vi "clone.vi"(0 "reference":refnum<class "Graphics.lvclass">, 5 "error in (no error)":errorcluster) -> (14 "reference out":refnum<class "Graphics.lvclass">, 15 "clonedObjectRef":refnum<class "Graphics.lvclass">, 19 "error out":errorcluster)   [LabVIEW 2014, in "Graphics.lvclass"]
doc: "Clopned the object"
uses:
  <resource>/Framework/Providers/Open_GDS/UML/Graphics_class/Graphics.lvclass
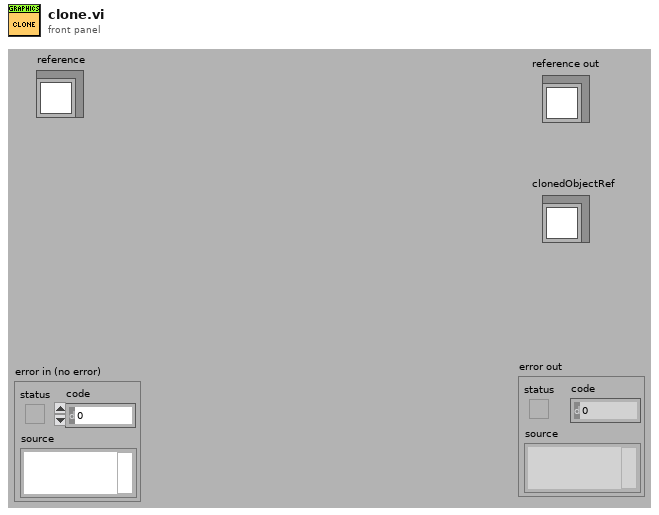
[diagram p1: front panel]
types:
  T1 = typedef "Graphics.lvclass/ObjectAttributes.ctl" = cluster{"drawColor":u32, "backgroundColor":u32, "font":T2, "fontType":T3, "picture":picture, "stroke":T4, "scaleX":dbl, "scaleY":dbl, "screenRef":refnum<vi>, "offsetX":dbl, "offsetY":dbl}
  T2 = typedef "Graphics.lvclass/FontType.ctl" = cluster{"Font Name:":string, "Size":i16, "Strikeout?":bool, "Italic?":bool, "Underline?":bool, "Outline?":bool, "Shadow?":bool, "Bold?":bool}
  T3 = typedef "Graphics.lvclass/LvFontType.ctl" = enum16{"User-specified Font", "Application Font", "System Font", "Dialog Font"}
  T4 = typedef "Graphics.lvclass/StrokeType.ctl" = enum16{"USE_DEFAULT", "SOLID", "DOTTED"}
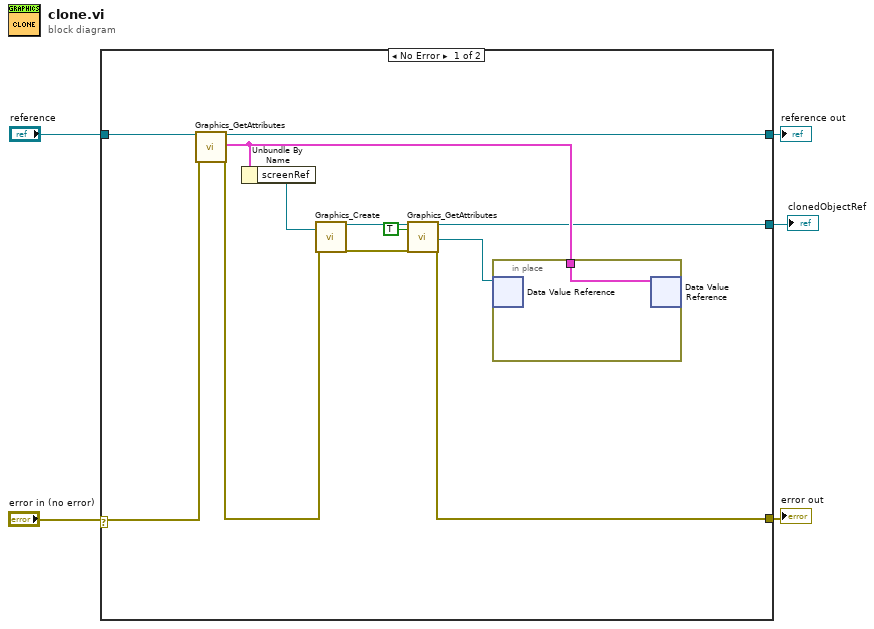
[diagram p0: block diagram]
diagram:
  n1 = case shown="No Error" "error in (no error)" {
    selector: "error in (no error)" -> [w15 w19]
    tunnel: "reference" -> [w17 w20]
    tunnel: [w7 w19] -> w4
    tunnel: [w16 w20] -> w3
    tunnel: [w6 _] -> w1
    frame No Error {
      n2 = call <resource>:"Graphics_GetAttributes.vi"("reference in"=w17, "error in (no error)"=w15) -> ("reference out"=w16:refnum<class "Graphics.lvclass">, "Data"=w8:T1, "error out"=w13:errorcluster)  [unwired: 1 in, 14 out]
      n3 = Unbundle By Name(w8) -> ("screenRef"=w14:refnum<vi>)
      n4 = call <resource>:"Graphics_Create.vi"("screenRef"=w14, "error in (no error)"=w13) -> ("reference out"=w12:refnum<class "Graphics.lvclass">, "error out"=w11:errorcluster)  [unwired: 1 in, 15 out]
      n5 = call <resource>:"Graphics_GetAttributes.vi"("reference in"=w12, "OnlyGetDvrReference(False)"=TRUE, "error in (no error)"=w11) -> ("reference out"=w6:refnum<class "Graphics.lvclass">, "DataRef"=w9:refnum<data-value>, "error out"=w7:errorcluster)  [unwired: 13 in, 1 out]
      n6 = in-place {
        in-place-border: w8 -> [w18]
        n7 = in-place-dvr #1(w9) -> ()  [unwired: 2 out]
        n8 = in-place-dvr #1(w18) -> ()  [unwired: 2 out]
      }
    }
    frame Error {
    }
  }
  "reference out" <- w3
  "error out" <- w4
  "clonedObjectRef" <- w1
